vi "IsExecutable.vi"(8 "Error In":errorcluster) -> (0 "Error Out":errorcluster, 3 "Executable?":bool)   [LabVIEW 2013, in "LV-Utilities.lvlib"]
doc: "This VI checks if the top-level application VI is running as an executabled (.exe)."
uses:
  LV-Utilities.lvlib
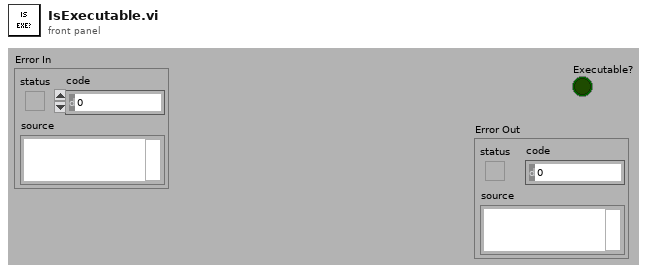
[diagram p1: front panel]
types:
  T1 = enum32{"invalid app kind", "Development System", "Run Time System", "Student Edition", "Embedded LabVIEW", "Evaluation", "Custom"}
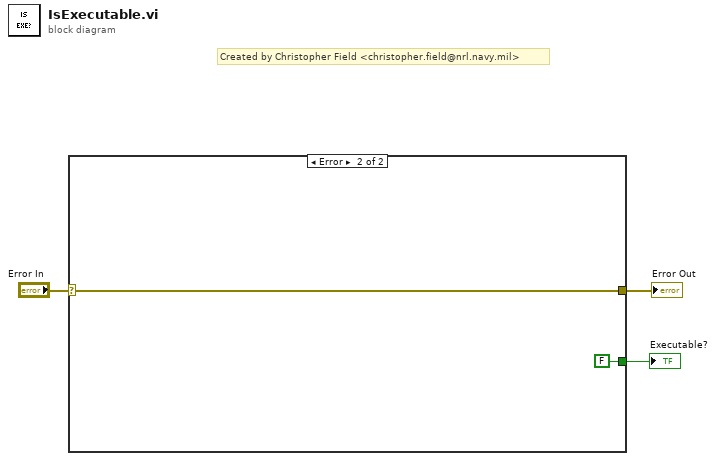
[diagram p0: block diagram]
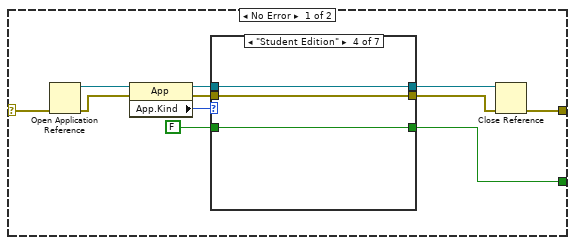
[diagram p2: hidden frame]
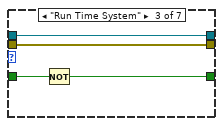
[diagram p5: hidden frame]
diagram:
  # "Created by Christopher Field <christopher.field@nrl.navy.mil>"
  n1 = case shown="Error" "Error In" {
    selector: "Error In" -> [w4 w38]
    tunnel: [w11 FALSE] -> w3
    tunnel: [w5 w38] -> w2
    frame No Error {
      n2 = Open Application Reference(8:w4) -> (0:w10:errorcluster, 3:w9:refnum<vi>)  [unwired: 3 in]
      n3 = property class="App"(reference=w9, error in=w10) -> (reference out=w13:refnum<vi>, error out=w8:errorcluster, "App.Kind"=w14:T1)
      n4 = case shown="\"Student Edition\"" w14 {
        tunnel: w13 -> [w17 w19 w24 w27 w30 w33 w36]
        tunnel: [w17 w19 w24 w27 w30 w33 w36] -> w7
        tunnel: [w16 w20 w22 w26 w29 w32 w35] -> w11
        tunnel: FALSE -> [w16 w20 w23 w26 w29 w32 w35]
        tunnel: w8 -> [w15 w18 w21 w25 w28 w31 w34]
        tunnel: [w15 w18 w21 w25 w28 w31 w34] -> w6
        frame "invalid app kind", Default {
        }
        frame "Development System" {
        }
        frame "Run Time System" {
          n5 = Not(x=w23) -> (.not. x?=w22:bool)
        }
        frame "Student Edition" {
        }
        frame "Embedded LabVIEW" {
        }
        frame "Evaluation" {
        }
        frame "Custom" {
        }
      }
      n6 = Close Reference(reference=w7, error in (no error)=w6) -> (error out=w5:errorcluster)
    }
    frame Error {
    }
  }
  "Error Out" <- w2
  "Executable?" <- w3
